vi "Receive Value.vi"(10 "Numeric":dbl, 11 "Abstraction in":refnum<class "Abstraction.lvclass">) -> (3 "Abstraction out":refnum<class "Abstraction.lvclass">)   [LabVIEW 2023, in "Abstraction.lvlib" / "Abstraction.lvclass"]
uses:
  Abstraction.lvclass
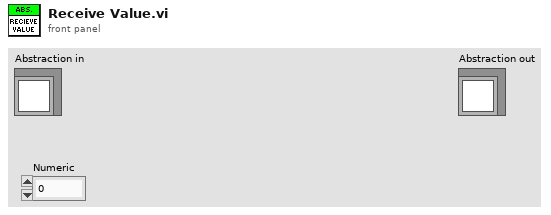
[diagram p1: front panel]
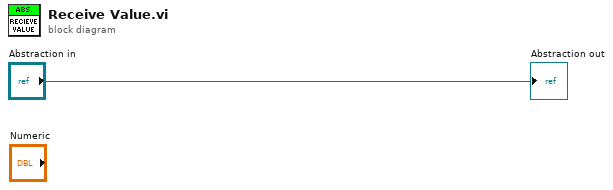
[diagram p0: block diagram]
diagram:
  "Abstraction out" <- "Abstraction in"
